vi "UDT_lowLevelControllerModule_lowLevelControllerPreRun.vi"() -> (3 "Unit Test Framework Results":T1)   [LabVIEW 2017]
doc: "Use this template to create a user-defined test VI. Define your test requirements and wire the results to the <b>Result (Test)</b> control. Do not modify the <b>Unit Test Framework Results</b> indicator."
uses:
  <vilib>/utf/common/utf_test_result_troll.ctl
  <vilib>/utf/common/utf_test_result.ctl
  <vilib>/utf/common/utf_test_result_failure.ctl
  <vilib>/utf/common/utf_test_comparison_operators.ctl
  <vilib>/utf/common/utf_vi_tag.ctl
  RT/LowLevelController/Queue/TypeDefs/queueFGVState.ctl
  RT/LowLevelController/Queue/TypeDefs/message.ctl
  <vilib>/Control Software Solutions Ltd/UTF Helper/SubVIs/UTF Variant Equals.vi
  <vilib>/Control Software Solutions Ltd/UTF Helper/Unit Test Helper.lvlib
  RT/LowLevelController/lowLevelController.lvlib
  <vilib>/utf/NI_UnitTestFramework.lvlib
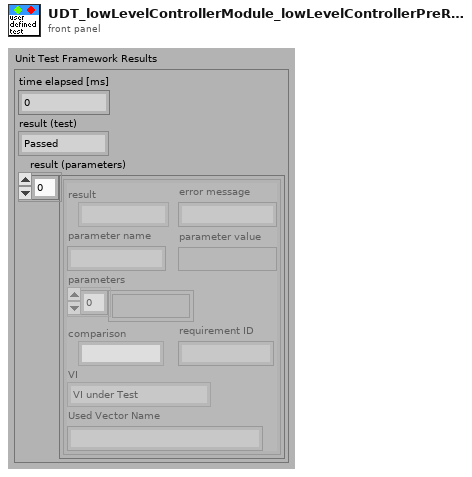
[diagram p1: front panel]
types:
  T1 = typedef "NI_UnitTestFramework.lvlib/utf_test_result_troll.ctl" = cluster{"time elapsed [ms]":u32, "result (test)":T2, "result (parameters)":T3[]}
  T2 = typedef "NI_UnitTestFramework.lvlib/utf_test_result.ctl" = enum16{"Passed", "Failed", "Error", "Skipped", "Not Processed"}
  T3 = typedef "NI_UnitTestFramework.lvlib/utf_test_result_failure.ctl" = cluster{"result":T2, "error message":string, "parameter name":string, "parameter value":variant, "parameters":variant[], "comparison":T4, "requirement ID":string, "VI":T5, "Used Vector Name":string}
  T4 = typedef "NI_UnitTestFramework.lvlib/utf_test_comparison_operators.ctl" = enum16{"=", "!=", ">", ">=", "<", "<=", "range", "symmetric tolerance", "asymmetric tolerance", "string contains", "string not contain", "array size", "string length", "array range", "by element", "array range (limit array)", "user-defined", "array contains", "array not contain", "vector length", "= (elm)", "!= (elm)", "= (case insensitive)", "!= (case insensitive)"}
  T5 = typedef "NI_UnitTestFramework.lvlib/utf_vi_tag.ctl" = enum16{"Setup VI", "VI under Test", "Teardown VI"}
  T6 = typedef "lowLevelController.lvlib/message.ctl" = cluster{"calling module":string, "message":string, "data":variant}
  T7 = typedef "lowLevelController.lvlib/queueFGVState.ctl" = enum16{"obtain", "enqueue low priority", "enqueue high priority", "dequeue", "release"}
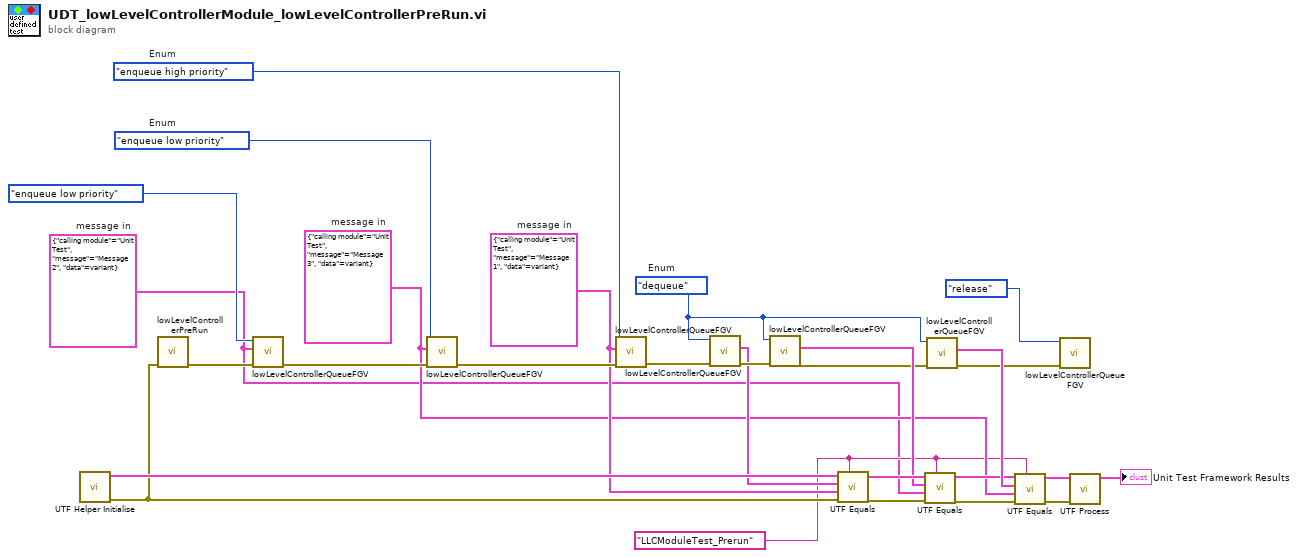
[diagram p0: block diagram]
diagram:
  w1 = T6 {"calling module"="Unit Test", "message"="Message 2", "data"=variant}  # message in
  w4 = "LLCModuleTest_Prerun"
  w13 = queueFGVState."dequeue"  # Enum
  w21 = T6 {"calling module"="Unit Test", "message"="Message 1", "data"=variant}  # message in
  w9 = T6 {"calling module"="Unit Test", "message"="Message 3", "data"=variant}  # message in
  w25 = queueFGVState."enqueue high priority"  # Enum
  w27 = queueFGVState."enqueue low priority"  # Enum
  n1 = call <vilib>:"UTF Helper Initialise.vi"() -> ("error out"=w22:errorcluster, "results array"=w23:T3[])  [unwired: 10 in]
  n2 = call "lowLevelControllerPreRun.vi"("error in (no error)"=w22) -> ("error out"=w28:errorcluster)  [unwired: 10 in]
  n3 = call "lowLevelControllerQueueFGV.vi"("error in (no error)"=w28, "message in"=w1, 11:queueFGVState."enqueue low priority") -> ("error out"=w26:errorcluster)  [unwired: 7 in, 1 out]
  n4 = call "lowLevelControllerQueueFGV.vi"("error in (no error)"=w26, "message in"=w9, 11:w27) -> ("error out"=w24:errorcluster)  [unwired: 7 in, 1 out]
  n5 = call "lowLevelControllerQueueFGV.vi"("error in (no error)"=w24, "message in"=w21, 11:w25) -> ("error out"=w20:errorcluster)  [unwired: 7 in, 1 out]
  n6 = call "lowLevelControllerQueueFGV.vi"("error in (no error)"=w20, 11:w13) -> ("error out"=w17:errorcluster, "message out"=w16:T6)  [unwired: 8 in]
  n7 = call "lowLevelControllerQueueFGV.vi"("error in (no error)"=w17, 11:w13) -> ("error out"=w14:errorcluster, "message out"=w15:T6)  [unwired: 8 in]
  n8 = call-poly <vilib>:"UTF Equals.vi"("Parameter Name"=w4, "error in (no error)"=w22, "Test Value"=w21, "Input"=w16, "Input Results"=w23) -> ("error out"=w19:errorcluster, "Output Results"=w18:T3[])  [unwired: 5 in]
  n9 = call-poly <vilib>:"UTF Equals.vi"("Parameter Name"=w4, "error in (no error)"=w19, "Test Value"=w1, "Input"=w15, "Input Results"=w18) -> ("error out"=w10:errorcluster, "Output Results"=w11:T3[])  [unwired: 5 in]
  n10 = call "lowLevelControllerQueueFGV.vi"("error in (no error)"=w14, 11:w13) -> ("error out"=w6:errorcluster, "message out"=w12:T6)  [unwired: 8 in]
  n11 = call-poly <vilib>:"UTF Equals.vi"("Parameter Name"=w4, "error in (no error)"=w10, "Test Value"=w9, "Input"=w12, "Input Results"=w11) -> ("error out"=w7:errorcluster, "Output Results"=w8:T3[])  [unwired: 5 in]
  n12 = call "lowLevelControllerQueueFGV.vi"("error in (no error)"=w6, 11:queueFGVState."release" ("Enum")) -> ()  [unwired: 8 in, 2 out]
  n13 = call <vilib>:"UTF Process.vi"("error in (no error)"=w7, "results array"=w8) -> ("Unit Test Framework Results"=→"Unit Test Framework Results":T1)  [unwired: 9 in]
